vi "SVL AC & DC Level (Time) (N Ch).vi"(0 "scaled signals in [EU]":waveform(dbl)[](array[waveform]), 2 "window":u16(ring)=8 items=["None ", "Hanning", "Hamming", "Blackman-Harris", "Exact Blackman", "Blackman", "Flat Top", "4 Term B-Harris ", "7 Term B-Harris", "Low Sidelobe"], 5 "error in (no error)":errorcluster) -> (12 "unit labels":string[](array[string]), 14 "AC signals [EU]":waveform(dbl)[](array[waveform]), 15 "AC levels [EU rms]":dbl[](array[numeric]) format="%.8f", 16 "DC signals [EU]":waveform(dbl)[](array[waveform]), 17 "DC levels [EU]":dbl[](array[numeric]) format="%0.2f", 19 "error out":errorcluster)   [LabVIEW 2017]
doc: "Computes the AC level and DC level of a signal. Wire data to the <B>scaled signal [EU]</B> input to determine the polymorphic instance to use or manually select the instance."
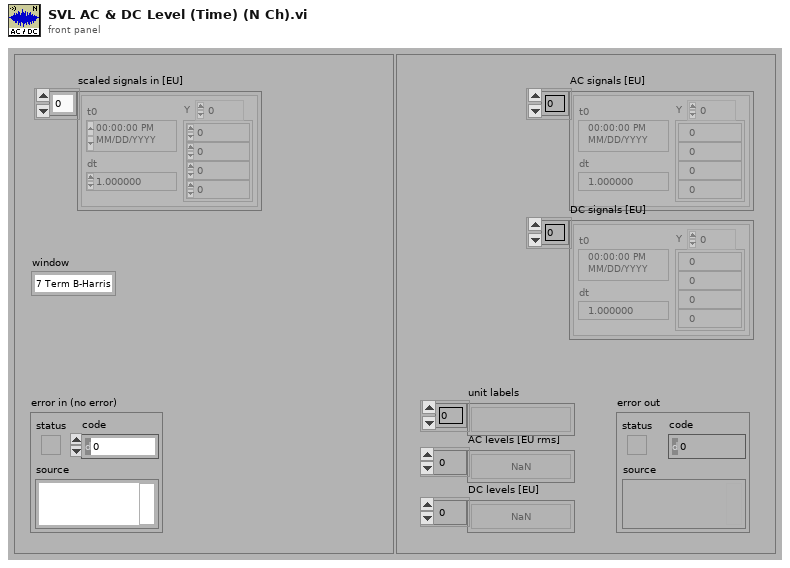
[diagram p1: front panel]
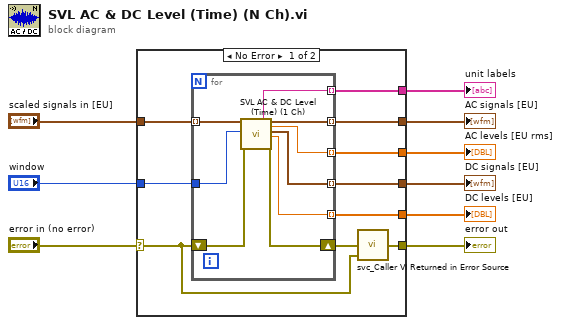
[diagram p0: block diagram]
diagram:
  n1 = case shown="No Error" "error in (no error)" {
    selector: "error in (no error)" -> [w11 w29]
    tunnel: [w19 _] -> w2
    tunnel: "window" -> [w13 _]
    tunnel: [w12 _] -> w8
    tunnel: "scaled signals in [EU]" -> [w17 _]
    tunnel: [w18 _] -> w6
    tunnel: [w14 w29] -> w4
    tunnel: [w16 _] -> w3
    tunnel: [w10 _] -> w1
    frame No Error {
      n2 = for {
        tunnel: [w22] -> w19 mode=indexing
        tunnel: [w21] -> w18 mode=indexing
        tunnel: w17 -> [w28] mode=indexing
        tunnel: [w23] -> w16 mode=indexing
        tunnel: w13 -> [w26]
        tunnel: [w27] -> w12 mode=indexing
        shift-right: [w24] -> w15
        shift-left: w11 -> [w25]
        tunnel: [w20] -> w10 mode=indexing
        n3 = call <vilib>:"SVL AC & DC Level (Time) (1 Ch).vi"("scaled signal [EU]"=w28, "window"=w26, "error in (no error)"=w25) -> ("unit label"=w20:string, "AC signal [EU]"=w27:waveform(dbl), "AC level [EU rms]"=w23:dbl, "DC signal [EU]"=w22:waveform(dbl), "DC level [EU]"=w21:dbl, "error out"=w24:errorcluster)  [unwired: 11 in]
      }
      n4 = call <vilib>:"svc_Caller VI Returned in Error Source.vi"("warning input to caller"=w11, "error in (no error)"=w15) -> ("error out"=w14:errorcluster)  [unwired: 3 in]
    }
    frame Error {
    }
  }
  "AC levels [EU rms]" <- w3
  "DC levels [EU]" <- w6
  "AC signals [EU]" <- w8
  "error out" <- w4
  "unit labels" <- w1
  "DC signals [EU]" <- w2
